vi "Revision Query.vi"(8 "error in (no error)":errorcluster, 11 "VISA resource name":refnum<visa-resource-name>) -> (0 "error out":errorcluster, 1 "Instrument Firmware Revision":string, 2 "Instrument Driver Revision":string, 3 "VISA resource name out":refnum<visa-resource-name>)   [LabVIEW 2015, in "Siglent SPD3000 Series.lvlib"]
doc: "Queries the current instrument firmware revision and instrument driver revision.\n\nRefer to the Readme file for detailed driver information including modification history."
uses:
  <instrlib>/Siglent SPD3000 Series/Siglent SPD3000 Series.lvlib
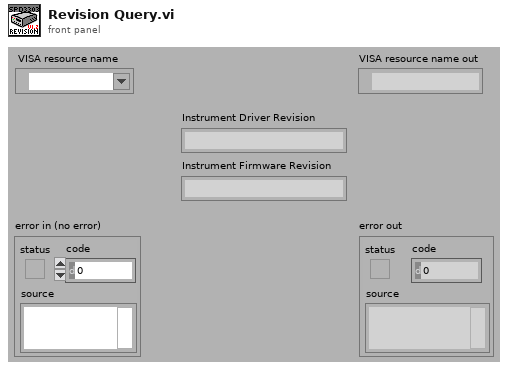
[diagram p1: front panel]
types:
  T1 = enum32{"invalid app kind", "Development System", "Run Time System", "Student Edition", "Embedded LabVIEW", "Evaluation", "Custom"}
  T2 = cluster{"Major":u16, "Minor":u16, "Fix":u16, "Build":u16}
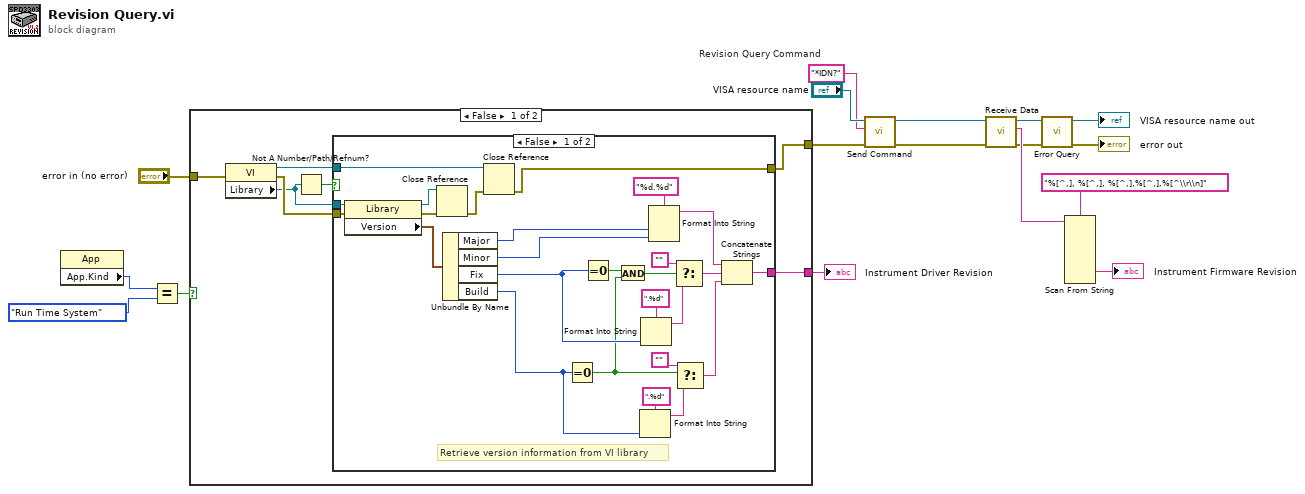
[diagram p0: block diagram]
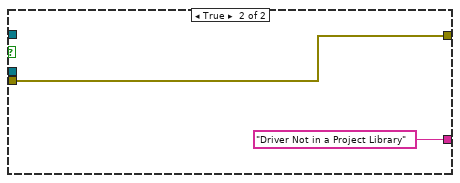
[diagram p2: hidden frame]
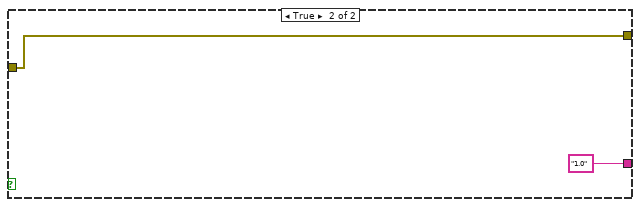
[diagram p3: hidden frame]
diagram:
  w16 = "*IDN?"  # Revision Query Command
  n1 = property class="App"() -> ("App.Kind"=w5:T1)  [unwired: 2 in, 2 out]
  n2 = Equal?(x=w5, y=T1."Run Time System" ("Application:Kind")) -> (x = y?=w6:bool)
  n3 = case shown="False" w6 {
    tunnel: [w21 "1.0"] -> w9
    tunnel: "error in (no error)" -> [w20 w53]
    tunnel: [w19 w53] -> w7
    frame False {
      n4 = property class="VI"(error in=w20) -> (reference out=w18:refnum<vi>, error out=w24:errorcluster, "Library"=w23:refnum<vi>)  [unwired: 1 in]
      n5 = Not A Number/Path/Refnum?(number/path/refnum=w23) -> (NaN/Path/Refnum?=w22:bool)
      n6 = case shown="False" w22 {
        tunnel: w18 -> [w47 _]
        tunnel: w24 -> [w32 w52]
        tunnel: [w27 w52] -> w19
        tunnel: [w26 "Driver Not in a Project Library"] -> w21
        tunnel: w23 -> [w25 _]
        frame False {
          # "Retrieve version information from VI library"
          n7 = property class="Library"(reference=w25, error in=w32) -> (reference out=w49:refnum<vi>, error out=w50:errorcluster, "Version"=w46:T2)
          n8 = Close Reference(reference=w49, error in (no error)=w50) -> (error out=w48:errorcluster)
          n9 = Unbundle By Name(w46) -> ("Major"=w35:u16, "Minor"=w34:u16, "Fix"=w31:u16, "Build"=w33:u16)
          n10 = Close Reference(reference=w47, error in (no error)=w48) -> (error out=w27:errorcluster)
          n11 = Equal To 0?(x=w33) -> (x = 0?=w29:bool)
          n12 = Equal To 0?(x=w31) -> (x = 0?=w30:bool)
          n13 = And(x=w30, y=w29) -> (x .and. y?=w28:bool)
          n14 = Format Into String(format string=".%d", w33) -> (resulting string=w39:string)  [unwired: 2 in, 1 out]
          n15 = Format Into String(format string=".%d", w31) -> (resulting string=w43:string)  [unwired: 2 in, 1 out]
          n16 = Format Into String(format string="%d.%d", w35, w34) -> (resulting string=w41:string)  [unwired: 2 in, 1 out]
          n17 = Select(t="", s=w28, f=w43) -> (s? t:f=w40:string)
          n18 = Select(t="", s=w29, f=w39) -> (s? t:f=w36:string)
          n19 = Concatenate Strings(w41, w40, w36) -> (w26:string)
        }
        frame True {
        }
      }
    }
    frame True {
    }
  }
  "Instrument Driver Revision" <- w9
  n20 = call <instrlib>:"Send Command.vi"("error in (no error)"=w7, "Write Buffer (\"\")"=w16, "VISA resource name"="VISA resource name") -> ("error out"=w2:errorcluster, "VISA resource name out"=w3:refnum<visa-resource-name>)  [unwired: 7 in]
  n21 = call <instrlib>:"Receive Data.vi"("error in (no error)"=w2, "VISA resource name"=w3) -> ("error out"=w13:errorcluster, "Read Buffer"=w15:string, "VISA resource name out"=w12:refnum<visa-resource-name>)  [unwired: 6 in, 1 out]
  n22 = call <instrlib>:"Error Query.vi"("error in (no error)"=w13, "VISA resource name"=w12) -> ("error out"=→"error out":errorcluster, "VISA resource name out"=→"VISA resource name out":refnum<visa-resource-name>)  [unwired: 6 in, 2 out]
  n23 = Scan From String(format string="%[^,], %[^,], %[^,],%[^,],%[^\\r\\n]", input string=w15) -> (output 4=→"Instrument Firmware Revision":string)  [unwired: 11 in, 3 out]
